vi "get file.vi"(8 "error in (no error)":errorcluster, 11 "device_type in":refnum<class "device_type.lvclass">) -> (0 "error out":errorcluster, 1 "csv file":bool, 2 "selected path":path, 3 "device_type out":refnum<class "device_type.lvclass">)   [LabVIEW 2021, in "device_type.lvclass"]
uses:
  device_type.lvclass
  device_type.lvclass/device_type.ctl
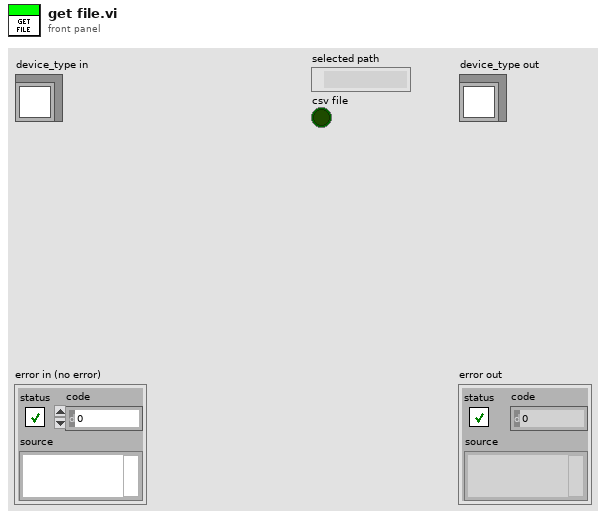
[diagram p1: front panel]
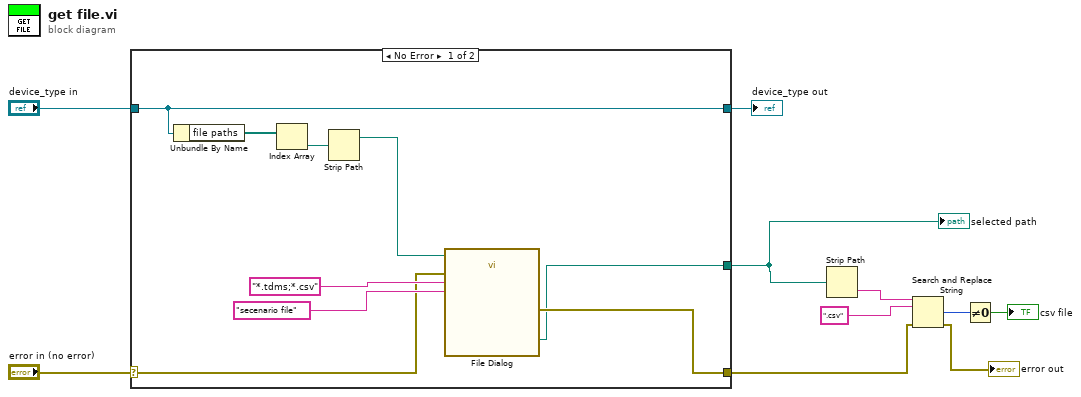
[diagram p0: block diagram]
diagram:
  n1 = case shown="No Error" "error in (no error)" {
    selector: "error in (no error)" -> [w16 w21]
    tunnel: [w15 w21] -> w3
    tunnel: [w13 w20] -> w8
    tunnel: "device_type in" -> [w13 w20]
    tunnel: [w14 _] -> w7
    frame No Error {
      n2 = Unbundle By Name(w13) -> ("file paths"=w12:path[])
      n3 = Index Array(array=w12) -> (element=w11:path)  [unwired: 1 in]
      n4 = Strip Path(path=w11) -> (stripped path=w17:path)  [unwired: 1 out]
      n5 = call "File Dialog"("start path"=w17, "error in"=w16, "pattern (all files)"="*.tdms;*.csv", "pattern label"="secenario file") -> ("selected path"=w14:path, "error out"=w15:errorcluster)  [unwired: 8 in, 2 out]
    }
    frame Error {
    }
  }
  "device_type out" <- w8
  "selected path" <- w7
  n6 = Strip Path(path=w7) -> (name=w6:string)  [unwired: 1 out]
  n7 = Search and Replace String(input string=w6, search string=".csv" ("format string"), error in=w3) -> (number of replacements=w4:i32, error out=→"error out":errorcluster)  [unwired: 5 in, 2 out]
  n8 = Not Equal To 0?(x=w4) -> (x != 0?=→"csv file":bool)
